vi "Get User Event from Event Name.vi"(8 "error in (no error)":errorcluster, 10 "Event Data":variant, 11 "Event Name (Quit)":string="Quit") -> (0 "error out":errorcluster, 3 "User Event out":refnum<user-event>)   [LabVIEW 2011]
doc: "This Vi will search for the <b>User Event</b> that exists in the <b>Event Data</b> Varient Repository based on the <b>Event Name</b>."
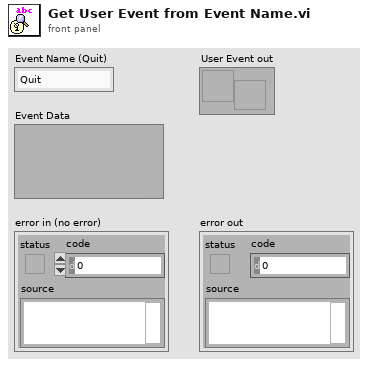
[diagram p1: front panel]
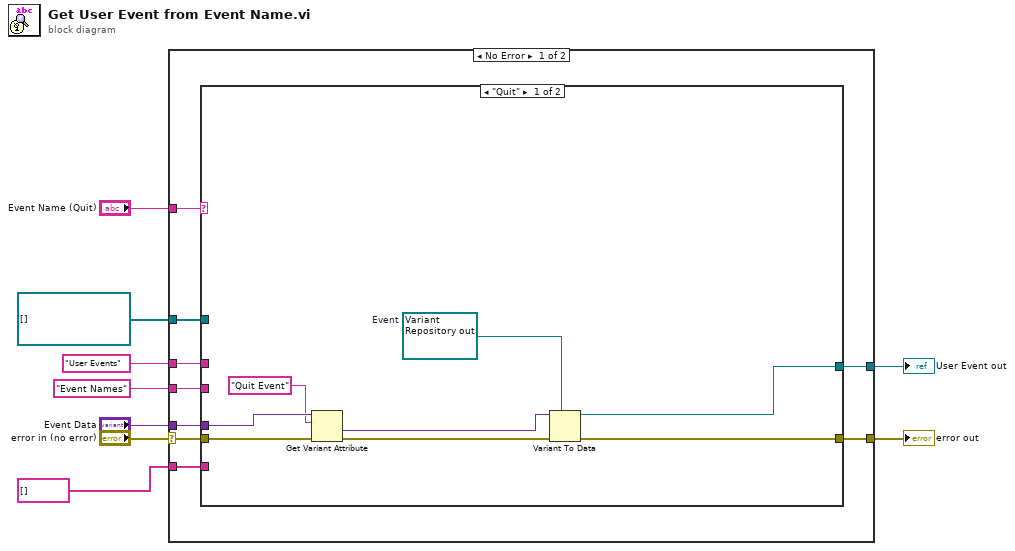
[diagram p0: block diagram]
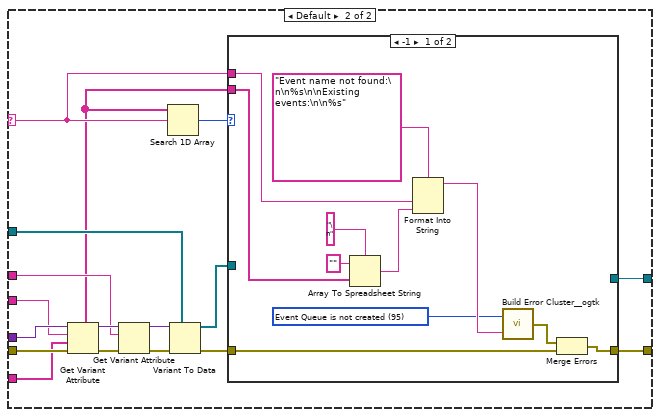
[diagram p2: hidden frame]
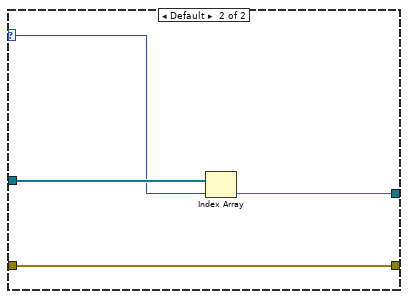
[diagram p3: hidden frame]
diagram:
  n1 = case shown="No Error" "error in (no error)" {
    selector: "error in (no error)" -> [w12 w59]
    tunnel: [w18 _] -> w9
    tunnel: refnum<user-event>[] [] -> [w17 _]
    tunnel: "Event Data" -> [w16 _]
    tunnel: "Event Names" ("Tag") -> [w15 _]
    tunnel: "User Events" ("Tag") -> [w14 _]
    tunnel: [w13 w59] -> w4
    tunnel: "Event Name (Quit)" -> [w11 _]
    tunnel: string[] [] -> [w10 _]
    frame No Error {
      n2 = case shown="\"Quit\"" w11 {
        selector: w11 -> [_ w37]
        tunnel: [w25 w43] -> w18
        tunnel: w17 -> [_ w41]
        tunnel: w16 -> [w23 w35]
        tunnel: w15 -> [_ w34]
        tunnel: w14 -> [_ w30]
        tunnel: [w24 w38] -> w13
        tunnel: w12 -> [w21 w36]
        tunnel: w10 -> [_ w33]
        frame "Quit" {
          w26 = refnum<user-event> refnum  # Event
          n3 = Get Variant Attribute(Variant=w23, name="Quit Event" ("Tag"), error in=w21) -> (value=w20:variant, error out=w19:errorcluster)  [unwired: 1 in, 2 out]
          n4 = Variant To Data(error in=w19, type=w26, Variant=w20) -> (data=w25:refnum<user-event>, error out=w24:errorcluster)
        }
        frame Default {
          n5 = Get Variant Attribute(Variant=w35, name=w34, default value (empty Variant)=w33, error in=w36) -> (duplicate Variant=w31:variant, value=w29:string[], error out=w32:errorcluster)  [unwired: 1 out]
          n6 = Get Variant Attribute(Variant=w31, name=w30, error in=w32) -> (value=w28:variant, error out=w27:errorcluster)  [unwired: 1 in, 2 out]
          n7 = Search 1D Array(1D array=w29, element=w37) -> (index of element=w40:i32)  [unwired: 1 in]
          n8 = Variant To Data(error in=w27, type=w41, Variant=w28) -> (data=w42:refnum<user-event>[], error out=w39:errorcluster)
          n9 = case shown="-1" w40 {
            selector: w40 -> [_ w56]
            tunnel: [_ w58] -> w43
            tunnel: w42 -> [_ w57]
            tunnel: w39 -> [w53 w55]
            tunnel: [w52 w55] -> w38
            tunnel: w29 -> [w46 _]
            tunnel: w37 -> [w47 _]
            frame -1 {
              w44 = 95 items=["No error", "Argument error", "Memory is full", "Out of zone", "End of file", "File already open", "Generic file I/O error", "File not found", "File permission error", "Disk is full", "Duplicate path", "Too many files open", "System feature not enabled", "Resource file not found", "Cannot add resource", "Resource not found", "Image not found", "Image memory error", "Pen does not exist", "Config type invalid", "Config token not found", "Config parse error", "Config memory error", "Bad external code format", "Bad external code offset", "External code not present", "Null window", "Destroy window error", "Null menu", "Print aborted", "Bad print record", "Print driver error", "Windows error during printing", "Memory error during printing", "Print dialog error", "Generic print error", "Invalid device refnum", "Device not found", "Device parameter error", "Device unit error", "Cannot open device", "Device call aborted", "Generic error", "Cancelled by user", "Object ID too low", "Object ID too high", "Object not in heap", "Unknown heap", "Unknown object (invalid DefProc)", "Unknown object (DefProc not in table)", "Message out of range", "Invalid (null) method", "Unknown message", "Manager call not supported", "Bad address", "Network operation in progress", "Network operation timed out", "Connection is busy", "Network attribute not supported", "Network error", "Address in use", "System out of memory", "Connection aborted", "Connection refused", "Not connected", "Already connected", "Connection closed", "Initialization error (interapplication manager)", "Bad occurrence", "Wait on unbound occurrence handler", "Occurrence queue overflow", "Datalog type conflict", "Unused", "Unrecognized type (interapplication manager)", "Memory corrupt", "Failed to make temporary DLL", "Old CIN version", "Drag socket not found", "Failed to load drop-object", "Failed to register OLE object", "Failed to release OLE object", "Format specifier type mismatch", "Unknown format specifier", "Too few format specifiers", "Too many format specifiers", "Scan failed", "Newer CIN version", "Error converting to variant", "Runtime menu error", "Password tampered", "Variant attribute not found", "Incompatible variant data type", "Event data is not available", "Event Store is not present", "Occurrence is not found", "Event Queue is not created", "Event info is not available", "Refnum passed is NULL", "Error retrieving Class GUID", "Error retrieving CoClass GUID", "Error retrieving TypeLib GUID.", "Bad built application magic bytes.", "Specific driver is different from the specific driver associated with the Logical Name.", "There is no session opened to the class driver.", "Max Error", "MAX - Error with config objects", "MAX - Error loading configuration", "MAX - Group not supported"]
              n10 = Array To Spreadsheet String(delimiter (Tab)="\n", array=w46, 3:"" ("format string")) -> (spreadsheet string=w50:string)
              n11 = Format Into String(format string="Event name not found:\n\n%s\n\nExisting events:\n\n%s", w47, w50) -> (resulting string=w45:string)  [unwired: 2 in, 1 out]
              n12 = call <userlib>:"Build Error Cluster__ogtk.vi"("String to Prepend to source (\"\")"=w45, "code"=w44) -> ("error out"=w54:errorcluster)
              n13 = Merge Errors(w54, w53) -> (w52:errorcluster)
            }
            frame Default {
              n14 = Index Array(array=w57, index=w56) -> (element=w58:refnum<user-event>)
            }
          }
        }
      }
    }
    frame Error {
    }
  }
  "error out" <- w4
  "User Event out" <- w9
